vi "testUnflattenFrequencyFromXML.vi"() -> ()   [LabVIEW 2012, in "UnitsAndXML.lvlib"]
uses:
  <userlib>/Common/UnitsAndXML/UnitsAndXML.lvlib
  <userlib>/Common/UnitsAndXML/FlattenItemWithUnitToXML/FlattenFrequencyToXML/FrequencyUnit.ctl
  <userlib>/Common/UnitsAndXML/UnflattenItemWithUnitFromXML/UnflattenFrequencyFromXML/typeMethods/unflattenFrequencyFromXML_Array.vi
  <userlib>/Common/UnitsAndXML/UnflattenItemWithUnitFromXML/UnflattenFrequencyFromXML/typeMethods/unflattenFrequencyFromXML_Scalar.vi
panel:
  out "error out":errorcluster
  out "frequency":dbl[unit][](array[numeric])
  out "frequency":dbl[unit]
  in  "frequencyUnitInXML":T1
  in  "xmlStringArray":string="<frequency>15</frequency>\r\n<frequency>30</frequency>\r\n<frequency>45</frequency>\r\n<frequency>60</frequency>"
  in  "xmlStringScalar":string="<frequency>15</frequency>"
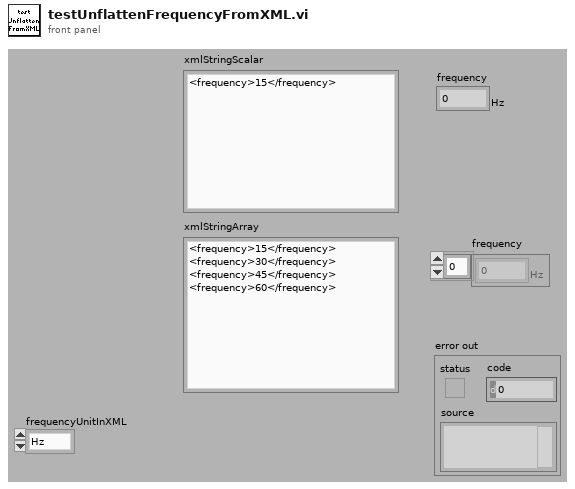
[diagram p1: front panel]
types:
  T1 = typedef "UnitsAndXML.lvlib/FrequencyUnit.ctl" = enum16{"Hz"}
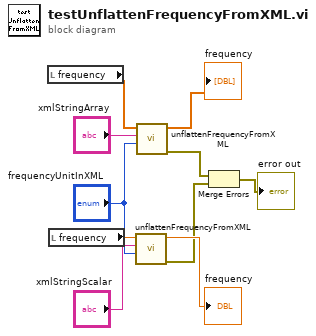
[diagram p0: block diagram]
diagram:
  n1 = local read "frequency"() -> (w3:dbl[unit][])
  n2 = local read "frequency"() -> (w9:dbl[unit])
  n3 = call-poly <userlib>:"unflattenFrequencyFromXML.vi"("frequencyUnitInXML"="frequencyUnitInXML", "xmlString"="xmlStringScalar", "frequencyForType"=w9) -> ("error out"=w5:errorcluster, "frequency"=→"frequency":dbl[unit])  [unwired: 7 in]
  n4 = call-poly <userlib>:"unflattenFrequencyFromXML.vi"("frequencyUnitInXML"="frequencyUnitInXML", "xmlString"="xmlStringArray", "frequencyForType"=w3) -> ("error out"=w6:errorcluster, "frequency"=→"frequency":dbl[unit][])  [unwired: 7 in]
  n5 = Merge Errors(w6, w5) -> (→"error out":errorcluster)
